vi "BlinkM WriteScriptLine.vi"(0 "Arduino Resource":T1={"VISA resource"="", "Board Type"=enum."Arduino Uno", "Connection Type"=enum."USB / Serial", "Bytes Per Packet (15)"=15}, 5 "Address (0)":u8, 7 "Script Line Parameters":T3 {"Argument 3" max=49; "Argument 2" max=49; "Argument 1" max=49; "BlinkM Command Code" max=49; "Line Duration (Ticks)" max=49; "Script Line (0 - 49)" max=49}, 11 "error in":errorcluster) -> (4 "Arduino Resource":T1={"VISA resource"="", "Board Type"=enum."Arduino Uno", "Connection Type"=enum."USB / Serial", "Bytes Per Packet (15)"=15}, 15 "error out":errorcluster)   [LabVIEW 2011, in "LabVIEW Interface for Arduino.lvlib"]
doc: "Write a line to the user editable script stored on the BlinkM.s"
uses:
  LabVIEW Interface for Arduino.lvlib
  Private/Type Defs/Arduino Resource.ctl
  Private/Type Defs/Board Type.ctl
  Private/Type Defs/BlinkM Script.ctl
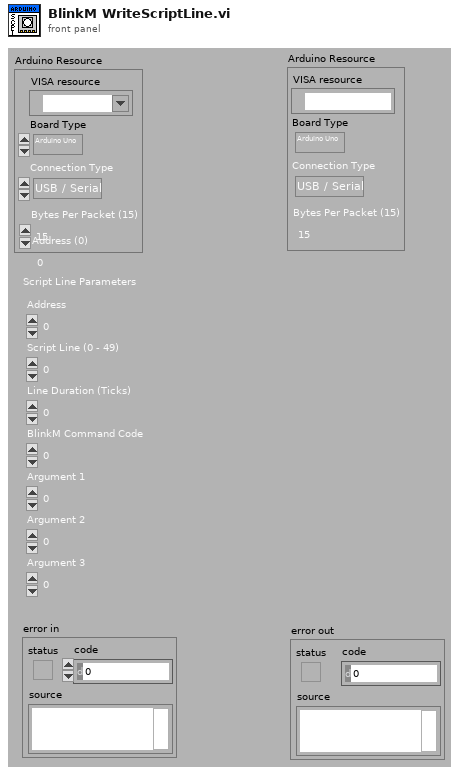
[diagram p1: front panel]
types:
  T1 = typedef "LabVIEW Interface for Arduino.lvlib/Arduino Resource.ctl" = cluster{"VISA resource":refnum<visa-resource-name>, "Board Type":T2, "Connection Type":enum8{"USB / Serial"}, "Bytes Per Packet (15)":u8}
  T2 = typedef "LabVIEW Interface for Arduino.lvlib/Board Type.ctl" = enum16{"Arduino Uno", "Dimuelanove w/Atmega 328", "Mega 2560", "Chipkit Uno32", "Chipkit Max32"}
  T3 = cluster{"Address":u8, "Script Line (0 - 49)":u8, "Line Duration (Ticks)":u8, "BlinkM Command Code":u8, "Argument 1":u8, "Argument 2":u8, "Argument 3":u8}
  T4 = typedef "LabVIEW Interface for Arduino.lvlib/BlinkM Script.ctl" = enum8{"User Script", "RGB", "White Flash", "Red Flash", "Green Flash", "Blue Flash", "Cyan Flash", "Magenta Flash", "Yellow Flash", "Black", "Hue Cycle", "Mood Light", "Virtual Candle", "Water Reflections", "Old Neon", "The Seasons", "Thunderstorm", "Stop Light", "Morse Code S.O.S"}
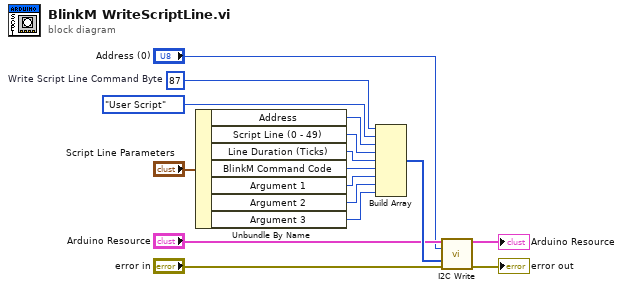
[diagram p0: block diagram]
diagram:
  w14 = u8 87  # Write Script Line Command Byte
  n1 = Unbundle By Name("Script Line Parameters") -> ("Address"=w10:u8, "Script Line (0 - 49)"=w9:u8, "Line Duration (Ticks)"=w8:u8, "BlinkM Command Code"=w7:u8, "Argument 1"=w6:u8, "Argument 2"=w5:u8, "Argument 3"=w4:u8)
  n2 = Build Array(w14, BlinkM_Script."User Script" ("BlinkM Script"), w10, w9, w8, w7, w6, w5, w4) -> (w13:u8[])
  n3 = call "I2C Write.vi"("Arduino Resource"="Arduino Resource", "Address (0)"="Address (0)", "I2C Data Bytes"=w13, "error in"="error in") -> ("Arduino Resource"=→"Arduino Resource":T1, "error out"=→"error out":errorcluster)  [unwired: 10 in]
